vi "Get Channel List.vi"(8 "error in (no error)":errorcluster, 9 "Control Value":u16, 10 "Control Reference":refnum<vi>, 11 "Hot And Cold Source Unit View in":refnum<class "Hot And Cold Source Unit View.lvclass">) -> (0 "error out":errorcluster, 3 "Hot And Cold Source Unit View out":refnum<class "Hot And Cold Source Unit View.lvclass">)   [LabVIEW 2013, in "Hot And Cold Source Unit View.lvlib" / "Hot And Cold Source Unit View.lvclass"]
uses:
  Hot And Cold Source Unit View.lvclass
  Hot And Cold Source Unit View.lvclass/Hot And Cold Source Unit View.ctl
  Common/Control Reference/Control Reference.lvlib
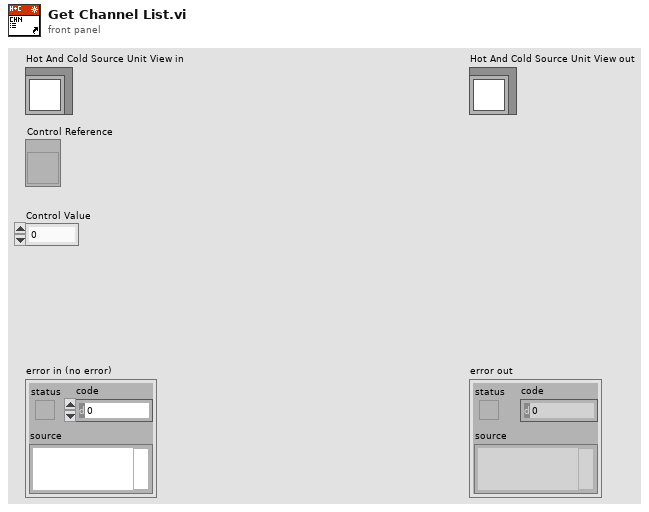
[diagram p1: front panel]
types:
  T1 = enum8{"Enabled", "Disabled", "Disabled and Grayed Out"}
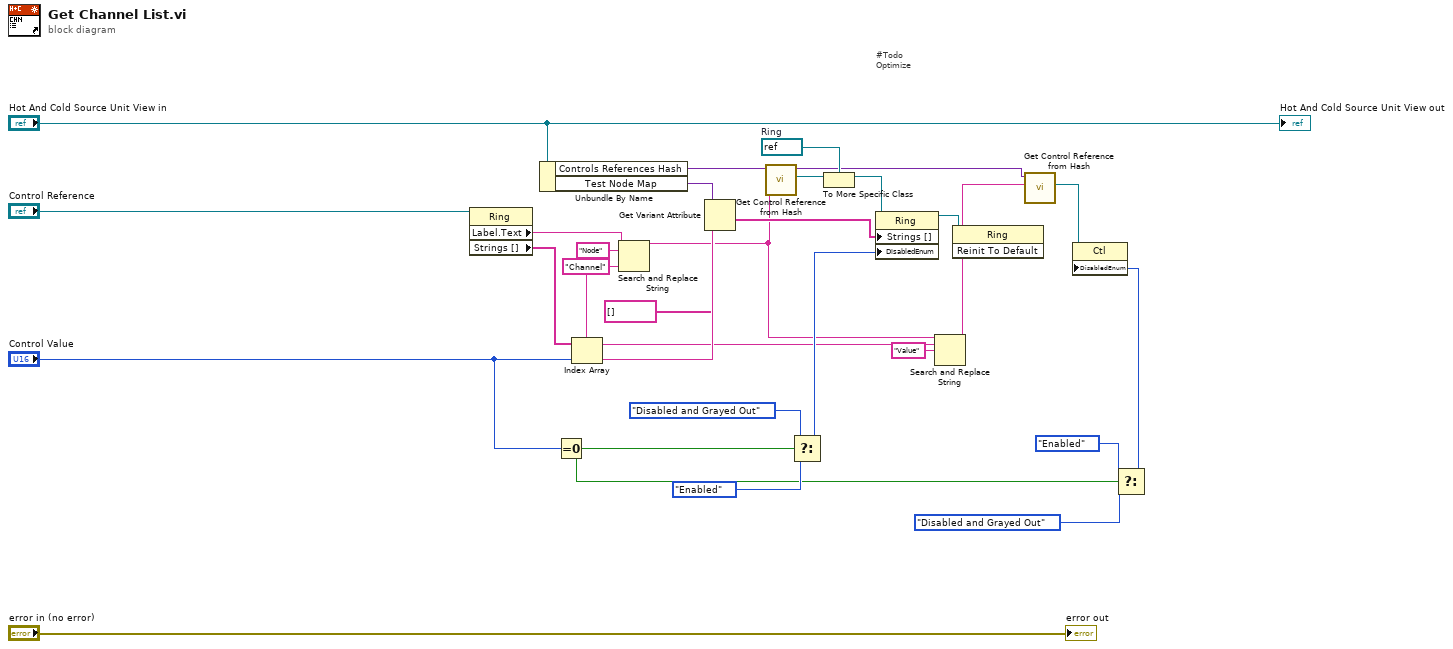
[diagram p0: block diagram]
diagram:
  w19 = refnum<vi> refnum  # Ring
  w9 = "Channel" ("replace string (\"\")")
  # "#Todo\nOptimize"
  n1 = property class="Ring"(reference="Control Reference") -> ("Label.Text"=w26:string, "Strings []"=w23:string[])  [unwired: 1 in, 2 out]
  n2 = Unbundle By Name("Hot And Cold Source Unit View in") -> ("Controls References Hash"=w27:variant, "Test Node Map"=w24:variant)
  n3 = Equal To 0?(x="Control Value") -> (x = 0?=w2:bool)
  n4 = Index Array(array=w23, index="Control Value") -> (element=w22:string)
  n5 = Search and Replace String(input string=w26, search string="Node", replace string=w9) -> (result string=w10:string)  [unwired: 5 in, 3 out]
  n6 = Get Variant Attribute(Variant=w24, name=w22, default value (empty Variant)=string[] []) -> (value=w17:string[])  [unwired: 1 in, 3 out]
  n7 = call "Get Control Reference from Hash.vi"("control label"=w10, "controls references hash"=w27) -> ("control reference"=w21:refnum<vi>, "duplicated controls references hash"=w11:variant)  [unwired: 6 in, 2 out]
  n8 = Select(t=T1."Disabled and Grayed Out" ("Disabled"), s=w2, f=T1."Enabled" ("Disabled")) -> (s? t:f=w13:T1)
  n9 = To More Specific Class(target class=w19, reference=w21) -> (specific class reference=w20:refnum<vi>)  [unwired: 1 in, 1 out]
  n10 = property class="Ring"(reference=w20, "Strings []"=w17, "DisabledEnum"=w13) -> (reference out=w1:refnum<vi>)  [unwired: 1 in, 1 out]
  n11 = Search and Replace String(input string=w10, search string=w9, replace string="Value" ("replace string (\"\")")) -> (result string=w6:string)  [unwired: 5 in, 3 out]
  n12 = invoke class="Ring" method="Reinit To Default"(reference=w1) -> ()  [unwired: 2 in, 3 out]
  n13 = call "Get Control Reference from Hash.vi"("control label"=w6, "controls references hash"=w11) -> ("control reference"=w7:refnum<vi>)  [unwired: 6 in, 3 out]
  n14 = Select(t=T1."Enabled" ("Disabled"), s=w2, f=T1."Disabled and Grayed Out" ("Disabled")) -> (s? t:f=w3:T1)
  n15 = property class="Ctl"(reference=w7, "DisabledEnum"=w3) -> ()  [unwired: 1 in, 2 out]
  "error out" <- "error in (no error)"
  "Hot And Cold Source Unit View out" <- "Hot And Cold Source Unit View in"
